vi "Radians_to_Degrees.vi"() -> ()   [LabVIEW 2020]
panel:
  out "Radians":dbl
  in  "Degrees":dbl
  out "Degrees":dbl
  in  "Radians":dbl
  # "Radians to Degrees"
  # "Degrees to Radians"
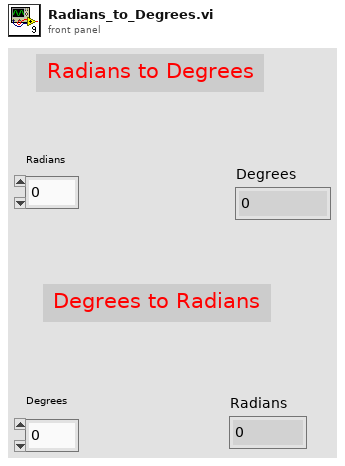
[diagram p1: front panel]
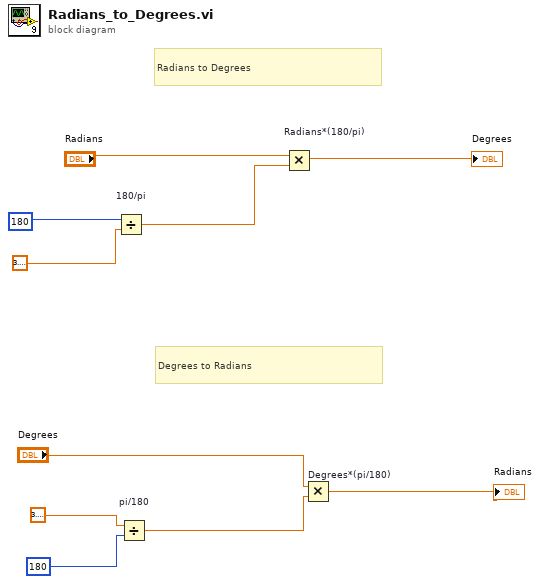
[diagram p0: block diagram]
diagram:
  # "Radians to Degrees"
  # "Degrees to Radians"
  n1 = Divide "180/pi"(x=180, y=3.141592653589793) -> (x/y=w7:dbl)
  n2 = Divide "pi/180"(x=3.141592653589793, y=180) -> (x/y=w1:dbl)
  n3 = Multiply "Radians*(180/pi)"(x="Radians", y=w7) -> (x*y=→"Degrees":dbl)
  n4 = Multiply "Degrees*(pi/180)"(x="Degrees", y=w1) -> (x*y=→"Radians":dbl)
